vi "Write Collected Data.vi"(8 "error in (no error)":errorcluster, 10 "Collected Data":refnum<class "AbstractData.lvclass">, 11 "AbstractCollector in":refnum<class "AbstractCollector.lvclass">) -> (0 "error out":errorcluster, 3 "AbstractCollector out":refnum<class "AbstractCollector.lvclass">)   [LabVIEW 2014, in "AbstractCollector.lvclass"]
uses:
  AbstractCollector.lvclass
  Model/Data/AbstractData/AbstractData.lvclass
  AbstractCollector.lvclass/AbstractCollector.ctl
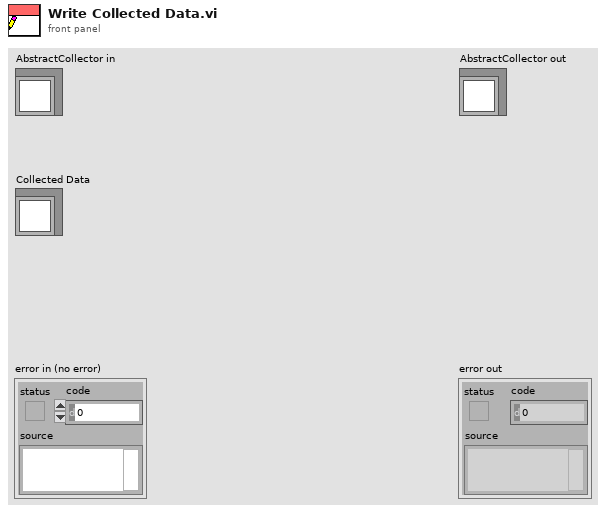
[diagram p1: front panel]
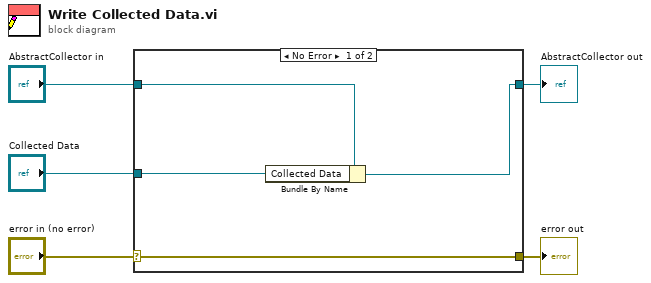
[diagram p0: block diagram]
diagram:
  n1 = case shown="No Error" "error in (no error)" {
    selector: "error in (no error)" -> [w9 w10]
    tunnel: [w9 w10] -> w4
    tunnel: [w7 w11] -> w2
    tunnel: "AbstractCollector in" -> [w8 w11]
    tunnel: "Collected Data" -> [w6 _]
    frame No Error {
      n2 = Bundle By Name(cluster=w8, "Collected Data"=w6) -> (w7:refnum<class "AbstractCollector.lvclass">)
    }
    frame Error {
    }
  }
  "error out" <- w4
  "AbstractCollector out" <- w2
